vi "read_pdo_mapping.vi"(9 "data":u32, 10 "subind":u8, 11 "index":u16) -> (2 "data":u32, 3 "return":i16)   [LabVIEW 2011]
uses:
  canopen_dll_master.dll
panel:
  in  "data":cluster{"data":u32}
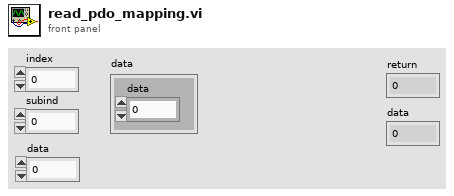
[diagram p1: front panel]
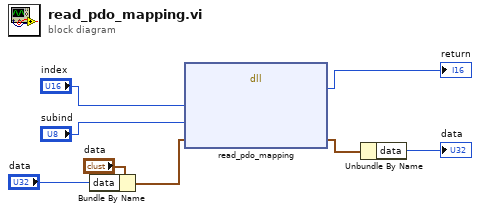
[diagram p0: block diagram]
diagram:
  n1 = Bundle By Name(cluster="data", "data"="data") -> (w3:cluster{"data":u32})
  n2 = dll-call lib="canopen_dll_master.dll" fn="read_pdo_mapping"("index"="index", "subind"="subind", "data"=w3) -> ("return type"=→"return":i16, "data"=w2:cluster{"data":u32})  [unwired: 5 in, 2 out]
  n3 = Unbundle By Name(w2) -> ("data"=→"data":u32)
